vi "Move XY to center.vi"() -> ()   [LabVIEW 2016, in "Drivers.lvlib" / "Agilis.lvlib"]
uses:
  Agilis.lvlib
panel:
  out "Total Steps":i32[](array[numeric])
  in  "Port":refnum<visa-resource-name>
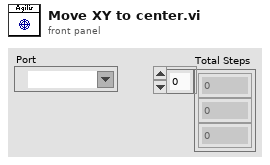
[diagram p1: front panel]
types:
  T1 = typedef "Drivers.lvlib/Agilis.lvlib/AgilisCmdLib Refnum.ctl" = refnum<k24>
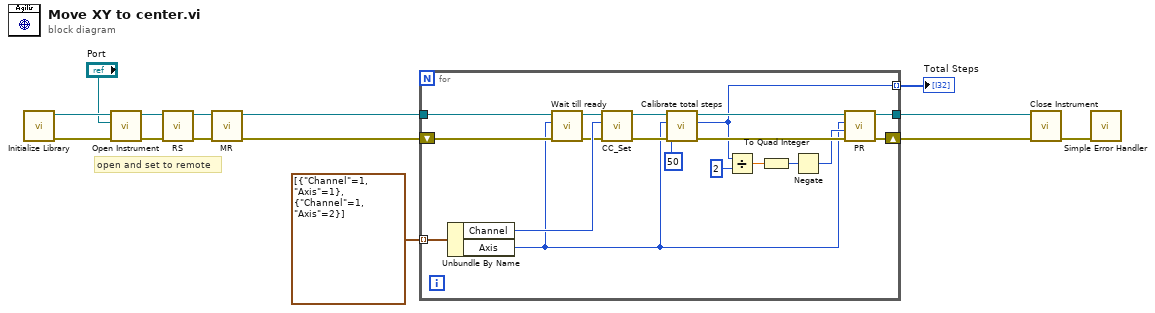
[diagram p0: block diagram]
diagram:
  # "open and set to remote"
  n1 = call "Initialize Library.vi"() -> ("error out"=w13:errorcluster, "Agilis out"=w14:T1)  [unwired: 10 in]
  n2 = call "Open Instrument.vi"("error in (no error)"=w13, "Device Key"="Port", "Agilis in"=w14) -> ("error out"=w4:errorcluster, "Agilis out"=w5:T1)  [unwired: 7 in]
  n3 = call "RS.vi"("error in (no error)"=w4, "Agilis in"=w5) -> ("error out"=w3:errorcluster, "Agilis out"=w2:T1)  [unwired: 8 in]
  n4 = call "MR.vi"("error in (no error)"=w3, "Agilis in"=w2) -> ("error out"=w12:errorcluster, "Agilis out"=w7:T1)  [unwired: 8 in]
  n5 = for {
    tunnel: cluster{"Channel":i32, "Axis":i32}[] [{"Channel"=1, "Axis"=1}, {"Channel"=1, "Axis"=2}] -> [w33] mode=indexing
    tunnel: w7 -> [w19]
    shift-right: [w27] -> w9
    shift-left: w12 -> [w18]
    tunnel: [w26] -> w6
    tunnel: [w25] -> w1 mode=indexing
    n6 = Unbundle By Name(w33) -> ("Channel"=w32:i32, "Axis"=w15:i32)
    n7 = call "Wait till ready.vi"("error in (no error)"=w18, "Axis Number"=w15, ".NET Refnum in"=w19) -> ("error out"=w17:errorcluster, ".NET Refnum out"=w16:T1)  [unwired: 7 in]
    n8 = call "CC_Set.vi"("error in (no error)"=w17, "Channel Number"=w32, "Agilis in"=w16) -> ("error out"=w30:errorcluster, "Agilis out"=w31:T1)  [unwired: 7 in]
    n9 = call "Calibrate total steps.vi"("error in (no error)"=w30, "Step Amplitude"=50, "Axis Number"=w15, "Agilis in"=w31) -> ("error out"=w28:errorcluster, "Total Steps"=w25:i32, "Agilis out"=w29:T1)  [unwired: 5 in]
    n10 = Divide(x=w25, y=2) -> (x/y=w23:dbl)
    n11 = To Quad Integer(1:w23) -> (0:w21:i64)
    n12 = Negate(x=w21) -> (-x=w20:i64)
    n13 = call "PR.vi"("error in (no error)"=w28, "Target Position"=w20, "Axis Number"=w15, "Agilis in"=w29) -> ("error out"=w27:errorcluster, "Agilis out"=w26:T1)  [unwired: 6 in]
  }
  "Total Steps" <- w1
  n14 = call "Close Instrument.vi"("error in (no error)"=w9, "Agilis in"=w6) -> ("error out"=w8:errorcluster)  [unwired: 9 in]
  n15 = call <vilib>:"Simple Error Handler.vi"("error in (no error)"=w8) -> ()  [unwired: 4 in, 5 out]
